vi "Sensor Interface.vi"(8 "error in (no error)":errorcluster, 10 "Queues":T1, 11 "UE Data Container":T2) -> (0 "error out":errorcluster)   [LabVIEW 2017]
doc: "Sensor Interface simulates a user making a deposit or withdrawal from the ATM.\n[Covers: UI4]"
uses:
  Shared Data/User Events/UE Data Container.ctl
  Error Handler/Controls/Error Data.ctl
  User Console/Controls/User Console - Transaction Enum.ctl
  Shared Data/Queues/Controls/Queues.ctl
  Controller/Controls/UI CMD.ctl
  Controller/Controls/Controller CMD.ctl
  Configuration/Controls/Config CMD.ctl
panel:
  in  "Funds Dispensed":bool
  in  "Deposit Received":bool
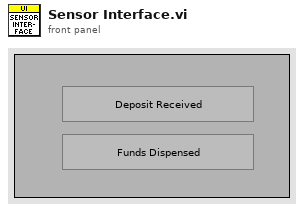
[diagram p1: front panel]
types:
  T1 = typedef "Queues.ctl" = cluster{"UI":refnum<queue>, "Controller":refnum<queue>, "Config":refnum<queue>, "User Console":refnum<queue>, "Display Console":refnum<queue>}
  T2 = typedef "UE Data Container.ctl" = cluster{"Stop UE":refnum<user-event>, "Error UE":refnum<user-event>, "Deposit Change":refnum<user-event>, "Funds Change":refnum<user-event>, "Card Reader Change":refnum<user-event>, "Transaction Change":refnum<user-event>, "Keypad Screen Change":refnum<user-event>}
  T3 = enum8{"Enabled", "Disabled", "Disabled and Grayed Out"}
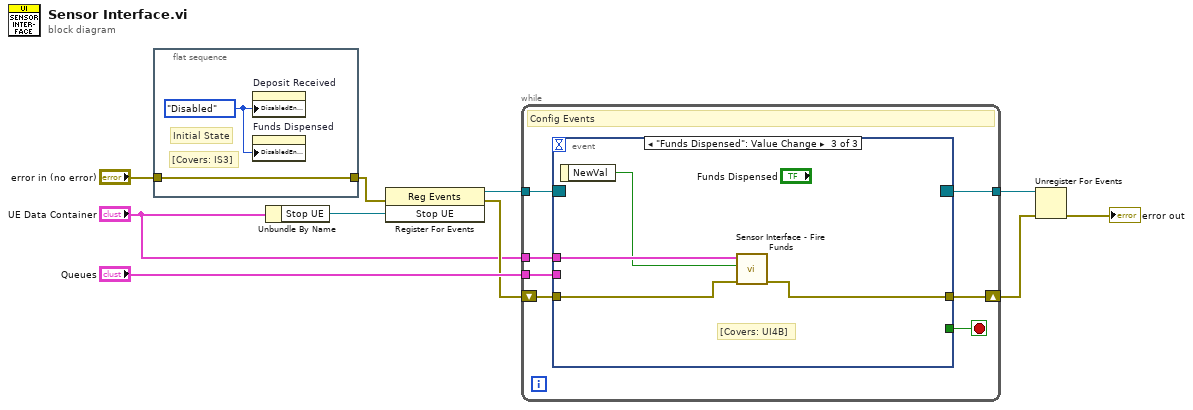
[diagram p0: block diagram]
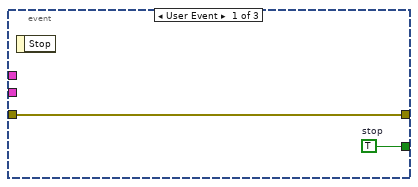
[diagram p2: hidden frame]
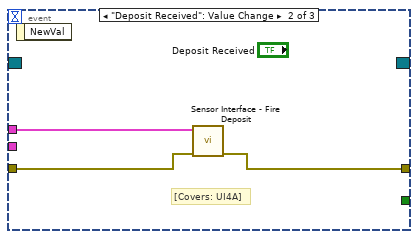
[diagram p3: hidden frame]
diagram:
  n1 = flat-sequence {
    tunnel: "error in (no error)" -> [w12]
    tunnel: [w12] -> w1
    frame #0 {
      w11 = T3."Disabled" ("Disabled")
      # "[Covers: IS3]"
      # "Initial State"
      n2 = property on="Deposit Received" class="Bool"("DisabledEnum"=w11) -> ()  [unwired: 2 in, 2 out]
      n3 = property on="Funds Dispensed" class="Bool"("DisabledEnum"=w11) -> ()  [unwired: 2 in, 2 out]
    }
  }
  n4 = Unbundle By Name("UE Data Container") -> ("Stop UE"=w10:refnum<user-event>)
  n5 = register-events(error in=w1, w10) -> (reference out=w9:refnum<event-registration>, error out=w5:errorcluster)  [unwired: 1 in]
  n6 = while {
    tunnel: w9 -> [w19]
    tunnel: [w18] -> w8
    tunnel: "Queues" -> [w16]
    shift-right: [w14] -> w7
    shift-left: w5 -> [w15]
    tunnel: "UE Data Container" -> [w13]
    stop <- w17 stop-if-true
    # "Config Events"
    n7 = event shown="[2] \"Funds Dispensed\": Value Change" {
      selector: w19 -> [_ _ _]
      dyn-events: [_ _ _] -> w18
      timeout: _ -> [_ _ _]
      tunnel: [w21 _ _] -> w17
      tunnel: w16 -> [_ _ _]
      tunnel: w15 -> [w20 w24 w27]
      tunnel: [w20 w22 w26] -> w14
      tunnel: w13 -> [_ w23 w28]
      event User Event {
        w21 = TRUE  # stop
        n8 = event-data() -> ()  [unwired: 1 in, 1 out]
      }
      event "Deposit Received": Value Change {
        # "[Covers: UI4A]"
        n9 = event-data() -> ()  [unwired: 1 in, 1 out]
        n10 = call "Sensor Interface - Fire Deposit.vi"("error in (no error)"=w24, "UE Data Container"=w23) -> ("error out"=w22:errorcluster)  [unwired: 9 in]
      }
      event "Funds Dispensed": Value Change {
        # "[Covers: UI4B]"
        n11 = event-data() -> ("NewVal"=w25:bool)  [unwired: 1 in]
        n12 = call "Sensor Interface - Fire Funds.vi"("error in (no error)"=w27, "Funds Change"=w25, "UE Data Container"=w28) -> ("error out"=w26:errorcluster)  [unwired: 8 in]
      }
    }
  }
  n13 = Unregister For Events(event registration refnum=w8, error in=w7) -> (error out=→"error out":errorcluster)
